vi "Create Pattern Script(OM).vi"(8 "error in (no error)":errorcluster, 11 "Operation Mode in":T1) -> (0 "error out":errorcluster, 3 "OM string out":string)   [LabVIEW 2018, in "BML_Frame_Root.lvclass"]
uses:
  BML_Frame_Root.lvclass
  Config_Read/OperationMode.ctl
  Config_Read/Config_Read_BML.lvclass
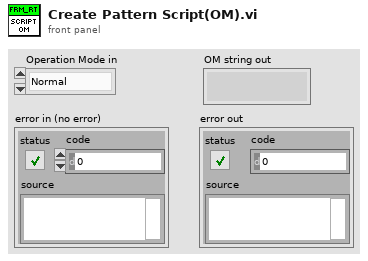
[diagram p1: front panel]
types:
  T1 = typedef "Config_Read_BML.lvclass/OperationMode.ctl" = enum8{"Normal", "ImmeEffect", "InitSlaveID", "LoadData"}
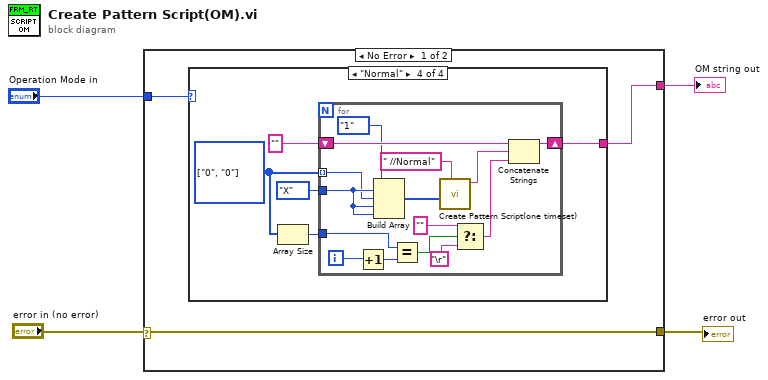
[diagram p0: block diagram]
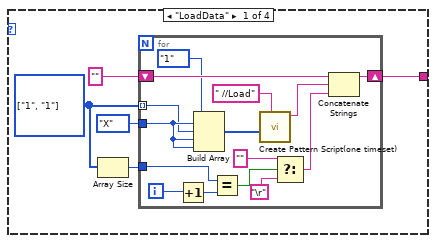
[diagram p2: hidden frame]
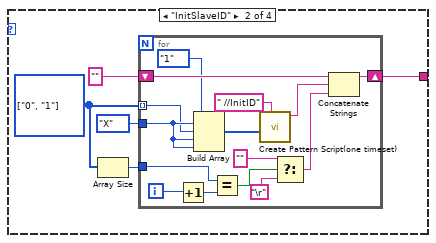
[diagram p3: hidden frame]
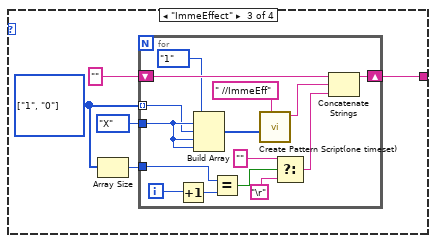
[diagram p4: hidden frame]
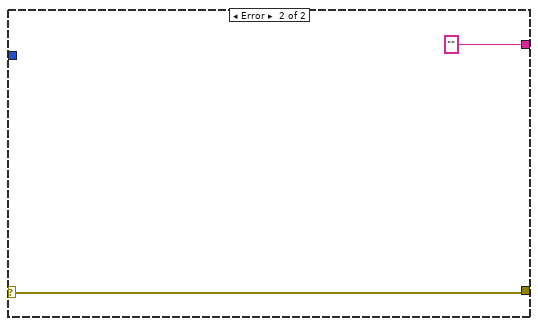
[diagram p5: hidden frame]
diagram:
  n1 = case shown="No Error" "error in (no error)" {
    selector: "error in (no error)" -> [w5 w88]
    tunnel: "Operation Mode in" -> [w7 _]
    tunnel: [w6 "" ("string out")] -> w2
    tunnel: [w5 w88] -> w1
    frame No Error {
      n2 = case shown="\"Normal\"" w7 {
        tunnel: [w11 w31 w51 w71] -> w6
        frame "LoadData" {
          w10 = enum16{"0", "1", "L", "H", "X", "V", "D", "M"}[] [enum."1", enum."1"] items=["0", "1", "L", "H", "X", "V", "D", "M"] ("PinState")
          n3 = Array Size(array=w10) -> (size(s)=w9:i32)
          n4 = for {
            tunnel: w10 -> [w15] mode=indexing
            shift-right: [w26] -> w11
            shift-left: "" ("string out") -> [w27]
            tunnel: w9 -> [w24]
            tunnel: enum16{"0", "1", "L", "H", "X", "V", "D", "M"}."X" ("element") -> [w18]
            i -> [w25]
            n5 = Increment(x=w25) -> (x+1=w23:i32)
            n6 = Build Array(enum16{"0", "1", "L", "H", "X", "V", "D", "M"}."1" ("element"), w18, w15, w18, w18) -> (w17:enum16{"0", "1", "L", "H", "X", "V", "D", "M"}[])
            n7 = Equal?(x=w24, y=w23) -> (x = y?=w22:bool)
            n8 = call "Create Pattern Script(one timeset).vi"("Notes"=" //Load", "PinState"=w17) -> ("string out"=w16:string)  [unwired: 9 in]
            n9 = Select(t="", s=w22, f="\r") -> (s? t:f=w19:string)
            n10 = Concatenate Strings(w27, w16, w19) -> (w26:string)
          }
        }
        frame "InitSlaveID" {
          w30 = enum16{"0", "1", "L", "H", "X", "V", "D", "M"}[] [enum."0", enum."1"] items=["0", "1", "L", "H", "X", "V", "D", "M"] ("PinState")
          n11 = Array Size(array=w30) -> (size(s)=w29:i32)
          n12 = for {
            tunnel: w30 -> [w35] mode=indexing
            shift-right: [w46] -> w31
            shift-left: "" ("string out") -> [w47]
            tunnel: w29 -> [w44]
            tunnel: enum16{"0", "1", "L", "H", "X", "V", "D", "M"}."X" ("element") -> [w38]
            i -> [w45]
            n13 = Increment(x=w45) -> (x+1=w43:i32)
            n14 = Build Array(enum16{"0", "1", "L", "H", "X", "V", "D", "M"}."1" ("element"), w38, w35, w38, w38) -> (w37:enum16{"0", "1", "L", "H", "X", "V", "D", "M"}[])
            n15 = Equal?(x=w44, y=w43) -> (x = y?=w42:bool)
            n16 = call "Create Pattern Script(one timeset).vi"("Notes"=" //InitID", "PinState"=w37) -> ("string out"=w36:string)  [unwired: 9 in]
            n17 = Select(t="", s=w42, f="\r") -> (s? t:f=w39:string)
            n18 = Concatenate Strings(w47, w36, w39) -> (w46:string)
          }
        }
        frame "ImmeEffect" {
          w50 = enum16{"0", "1", "L", "H", "X", "V", "D", "M"}[] [enum."1", enum."0"] items=["0", "1", "L", "H", "X", "V", "D", "M"] ("PinState")
          n19 = Array Size(array=w50) -> (size(s)=w49:i32)
          n20 = for {
            tunnel: w50 -> [w55] mode=indexing
            shift-right: [w66] -> w51
            shift-left: "" ("string out") -> [w67]
            tunnel: w49 -> [w64]
            tunnel: enum16{"0", "1", "L", "H", "X", "V", "D", "M"}."X" ("element") -> [w58]
            i -> [w65]
            n21 = Increment(x=w65) -> (x+1=w63:i32)
            n22 = Build Array(enum16{"0", "1", "L", "H", "X", "V", "D", "M"}."1" ("element"), w58, w55, w58, w58) -> (w57:enum16{"0", "1", "L", "H", "X", "V", "D", "M"}[])
            n23 = Equal?(x=w64, y=w63) -> (x = y?=w62:bool)
            n24 = call "Create Pattern Script(one timeset).vi"("Notes"=" //ImmeEff", "PinState"=w57) -> ("string out"=w56:string)  [unwired: 9 in]
            n25 = Select(t="", s=w62, f="\r") -> (s? t:f=w59:string)
            n26 = Concatenate Strings(w67, w56, w59) -> (w66:string)
          }
        }
        frame "Normal" {
          w70 = enum16{"0", "1", "L", "H", "X", "V", "D", "M"}[] [enum."0", enum."0"] items=["0", "1", "L", "H", "X", "V", "D", "M"] ("PinState")
          n27 = Array Size(array=w70) -> (size(s)=w69:i32)
          n28 = for {
            tunnel: w70 -> [w75] mode=indexing
            shift-right: [w86] -> w71
            shift-left: "" ("string out") -> [w87]
            tunnel: w69 -> [w84]
            tunnel: enum16{"0", "1", "L", "H", "X", "V", "D", "M"}."X" ("element") -> [w78]
            i -> [w85]
            n29 = Increment(x=w85) -> (x+1=w83:i32)
            n30 = Build Array(enum16{"0", "1", "L", "H", "X", "V", "D", "M"}."1" ("element"), w78, w75, w78, w78) -> (w77:enum16{"0", "1", "L", "H", "X", "V", "D", "M"}[])
            n31 = Equal?(x=w84, y=w83) -> (x = y?=w82:bool)
            n32 = call "Create Pattern Script(one timeset).vi"("Notes"=" //Normal", "PinState"=w77) -> ("string out"=w76:string)  [unwired: 9 in]
            n33 = Select(t="", s=w82, f="\r") -> (s? t:f=w79:string)
            n34 = Concatenate Strings(w87, w76, w79) -> (w86:string)
          }
        }
      }
    }
    frame Error {
    }
  }
  "error out" <- w1
  "OM string out" <- w2
